vi "GoodPID.vi"(7 "Enum":enum16{"Right Side", "Left Side"}(ring), 10 "Inputs":dbl[](array[numeric])) -> (2 "Back Motor Output":dbl, 3 "Front Motor Output":dbl, 4 "Left Side?":bool, 6 "Right Side?":bool)   [LabVIEW 2017]
uses:
  <vilib>/Rock Robotics/Network Tables/NT Write Number.vi
  <vilib>/addons/control/pid/pid.llb/PID (DBL).vi
  <vilib>/addons/control/pid/NI_PID_pid.lvlib
panel:
  out "PID Value":T1={"proportional gain (Kc)"=1.0, "integral time (Ti, min)"=0.01, "derivative time (Td, min)"=0.0} {"derivative time (Td, min)" format="%.3f"; "integral time (Ti, min)" format="%.3f"; "proportional gain (Kc)" format="%.3f"}
  in  "PID gains":T1={"proportional gain (Kc)"=1.0, "integral time (Ti, min)"=0.01, "derivative time (Td, min)"=0.0} {"derivative time (Td, min)" format="%.3f"; "integral time (Ti, min)" format="%.3f"; "proportional gain (Kc)" format="%.3f"}
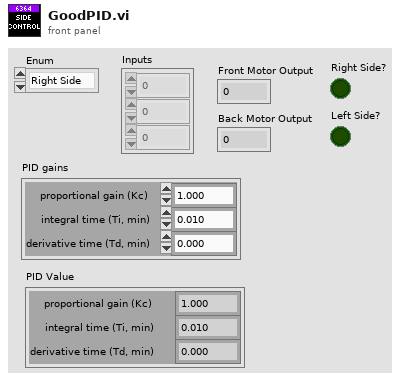
[diagram p1: front panel]
types:
  T1 = cluster{"proportional gain (Kc)":dbl, "integral time (Ti, min)":dbl, "derivative time (Td, min)":dbl}
  T2 = typedef "WPI_EncoderDevRef.ctl" = cluster{"DevStatus":errorcluster, "EncoderIndex":T3, "CounterIndex":T4, "DistancePerCount":dbl, "Decoding Type":T5}
  T3 = typedef "FPGA_EncoderIdx.ctl" = enum8{"Enc 0", "Enc 1", "Enc 2", "Enc 3", "Enc 4", "Enc 5", "Enc 6", "Enc 7", "Invalid"}
  T4 = typedef "FPGA_CounterCtrSystemIndex.ctl" = enum8{"Ctr 0", "Ctr 1", "Ctr 2", "Ctr 3", "Ctr 4", "Ctr 5", "Ctr 6", "Ctr 7", "Invalid"}
  T5 = typedef "WPI_EncoderType.ctl" = enum16{"1x", "2x", "4x"}
  T6 = typedef "WPI_MotorControlDeviceRef.ctl" = cluster{"DeviceStatus":errorcluster, "Type":T7, "PWM":cluster{"PWM Channel":T8, "DeadBand":T9}, "CAN":cluster{"Device Number":u8, "SetOutput VI Ref":variant, "GetOutput VI Ref":variant, "Enable VI Ref":variant, "Disable VI Ref":variant, "Data":variant}, "Invert":bool, "DIO PWM":cluster{"PWM \"Enable\" Channel":T8, "DIOChannel":T10, "PWM Rate":dbl}}
  T7 = typedef "WPI_MotorControlType.ctl" = enum16{"PWM", "CAN", "DIO PWM"}
  T8 = typedef "FPGA_DIOPWMChannel.ctl" = enum8{"PWM 0", "PWM 1", "PWM 2", "PWM 3", "PWM 4", "PWM 5", "PWM 6", "PWM 7", "PWM 8", "PWM 9", "PWM MXP 0", "PWM MXP 1", "PWM MXP 2", "PWM MXP 3", "PWM MXP 4", "PWM MXP 5", "PWM MXP 6", "PWM MXP 7", "PWM MXP 8", "PWM MXP 9", "Invalid"}
  T9 = typedef "WPI_PWMDeadband.ctl" = cluster{"Name":string, "maxPositivePwm":i32, "minPositivePwm":i32, "centerPwm":i32, "maxNegativePwm":i32, "minNegativePwm":i32, "angularRange":u16}
  T10 = typedef "FPGA_DIOChannel.ctl" = enum8{"DIO 0", "DIO 1", "DIO 2", "DIO 3", "DIO 4", "DIO 5", "DIO 6", "DIO 7", "DIO 8", "DIO 9", "DIO MXP 0", "DIO MXP 1", "DIO MXP 2", "DIO MXP 3", "DIO MXP 4", "DIO MXP 5", "DIO MXP 6", "DIO MXP 7", "DIO MXP 8", "DIO MXP 9", "DIO MXP 10", "DIO MXP 11", "DIO MXP 12", "DIO MXP 13", "DIO MXP 14", "DIO MXP 15", "SPI Port CS1", "SPI Port CS2", "SPI Port CS3", "SPI Port MISO", "SPI Port MOSI", "Invalid"}
  T11 = cluster{"MotorControlDevRef":T6, "MotorControlDevRef":T6}
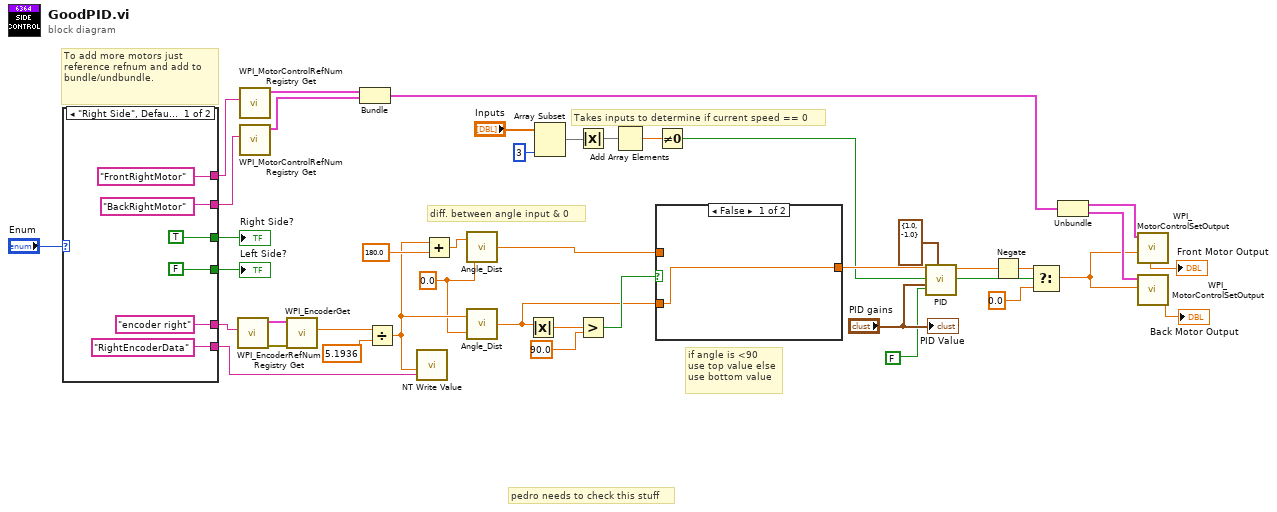
[diagram p0: block diagram]
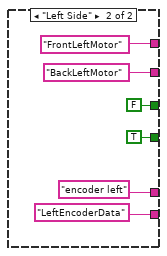
[diagram p3: hidden frame]
diagram:
  w23 = 0.0 ("TargetAngle")
  # "pedro needs to check this stuff"
  # "To add more motors just reference refnum and add to bundle/undbundle."
  # "if angle is <90\nuse top value else\nuse bottom value"
  # "diff. between angle input & 0"
  # "Takes inputs to determine if current speed == 0"
  n1 = case shown="\"Right Side\", Default" "Enum" {
    tunnel: ["FrontRightMotor" ("refnum name") "FrontLeftMotor" ("refnum name")] -> w41
    tunnel: ["BackRightMotor" ("refnum name") "BackLeftMotor" ("refnum name")] -> w38
    tunnel: ["encoder right" ("refnum name") "encoder left" ("refnum name")] -> w30
    tunnel: ["RightEncoderData" ("Name") "LeftEncoderData" ("Name")] -> w27
    tunnel: [TRUE ("Right Side?") FALSE ("Right Side?")] -> w2
    tunnel: [FALSE ("Left Side?") TRUE ("Left Side?")] -> w1
    frame "Right Side", Default {
    }
    frame "Left Side" {
    }
  }
  "Right Side?" <- w2
  "Left Side?" <- w1
  n2 = call <vilib>:"WPI_EncoderRefNum Registry Get.vi"("refnum name"=w30) -> ("error out"=w32:errorcluster, "EncoderDevRef"=w31:T2)  [unwired: 9 in]
  n3 = call <vilib>:"WPI_MotorControlRefNum Registry Get.vi"("refnum name"=w41) -> ("MotorControlDevRef"=w37:T6)  [unwired: 9 in, 1 out]
  n4 = call <vilib>:"WPI_MotorControlRefNum Registry Get.vi"("refnum name"=w38) -> ("MotorControlDevRef"=w36:T6)  [unwired: 9 in, 1 out]
  n5 = call <vilib>:"WPI_EncoderGet.vi"("error in (no error)"=w32, "EncoderDevRef"=w31) -> ("Distance"=w29:dbl)  [unwired: 4 in, 5 out]
  n6 = Bundle("MotorControlDevRef"=w37, "MotorControlDevRef"=w36) -> (w35:T11)  [unwired: 1 in]
  n7 = Divide(x=w29, y=5.1936) -> (x/y=w24:dbl)
  n8 = call-poly <vilib>:"NT Write Value.vi"("Numeric"=w24, "Name"=w27) -> ()  [unwired: 9 in, 1 out]
  n9 = Add(x=w24, y=180.0) -> (x+y=w25:dbl)
  n10 = call "Angle_Dist.vi"("TargetAngle"=w23, "CurrentAngle"=w25) -> ("Distance"=w18:dbl)
  n11 = call "Angle_Dist.vi"("TargetAngle"=w23, "CurrentAngle"=w24) -> ("Distance"=w19:dbl)
  n12 = Absolute Value(x=w19) -> (abs(x)=w22:dbl)
  n13 = Array Subset(array="Inputs", length=3) -> (w6:dbl[])  [unwired: 1 in]
  n14 = Absolute Value(x=w6) -> (abs(x)=w5:dbl[])
  n15 = Greater?(x=w22, y=90.0) -> (0:w20:bool)
  n16 = Add Array Elements(numeric array=w5) -> (sum=w4:dbl)
  n17 = case shown="False" w20 {
    tunnel: w19 -> [w54 _]
    tunnel: w18 -> [_ w55]
    tunnel: [w54 w55] -> w14
    frame False {
    }
    frame True {
    }
  }
  n18 = Not Equal To 0?(x=w4) -> (x != 0?=w3:bool)
  n19 = call-poly <vilib>:"PID.vi"("reinitialize? (F)"=FALSE, "output range"=cluster{"output high":dbl, "output low":dbl} {"output high"=1.0, "output low"=-1.0}, "PID gains"="PID gains", "setpoint"=w14) -> ("output"=w13:dbl)  [unwired: 6 in, 1 out]
  n20 = Negate(x=w13) -> (-x=w11:dbl)
  n21 = Select(t=w11, s=w3, f=0.0) -> (s? t:f=w10:dbl)
  n22 = Unbundle(w35) -> ("MotorControlDevRef"=w34:T6, "MotorControlDevRef"=w33:T6)
  n23 = call <vilib>:"WPI_MotorControlSetOutput.vi"("Output"=w10, "MotorControlDevRef"=w34) -> ("Motor Output"=→"Front Motor Output":dbl)  [unwired: 7 in, 2 out]
  n24 = call <vilib>:"WPI_MotorControlSetOutput.vi"("Output"=w10, "MotorControlDevRef"=w33) -> ("Motor Output"=→"Back Motor Output":dbl)  [unwired: 7 in, 2 out]
  "PID Value" <- "PID gains"
